vi "TestingStraight.vi"() -> ()   [LabVIEW 2016]
uses:
  <vilib>/Rock Robotics/WPI/Utilities/WPI_GetSetVariantRefNum.vi
panel:
  in  "Zero Yaw":bool
  in  "Config":T1={"Distance"=100.0, "MaxVelocity"=60.0, "MaxAccel"=50.0, "InitialVelocity"=0.0, "FinalVelocity"=0.0}
  out "Outputs":cluster{dbl, dbl, "Turn":dbl}(graph)
  in  "Go":bool
  in  "Go Backwards":bool
  out "Vel":cluster{dbl, "vel":dbl}(graph)
  out "Pos":cluster{dbl, "pos":dbl}(graph)={50.0, "pos"=48.31556625}
  in  "Linear Constants":T2={"FF"=0.0066, "AFF"=0.0018, "PID gains"={"P"=0.07, "I"=0.0, "D"=0.0}} {"PID gains"."D" format="%.3f"; "PID gains"."I" format="%.3f"; "PID gains"."P" format="%.3f"}
  # "MAKE DEFAULT"
  # ".009"
  # ".002"
  # ".07"
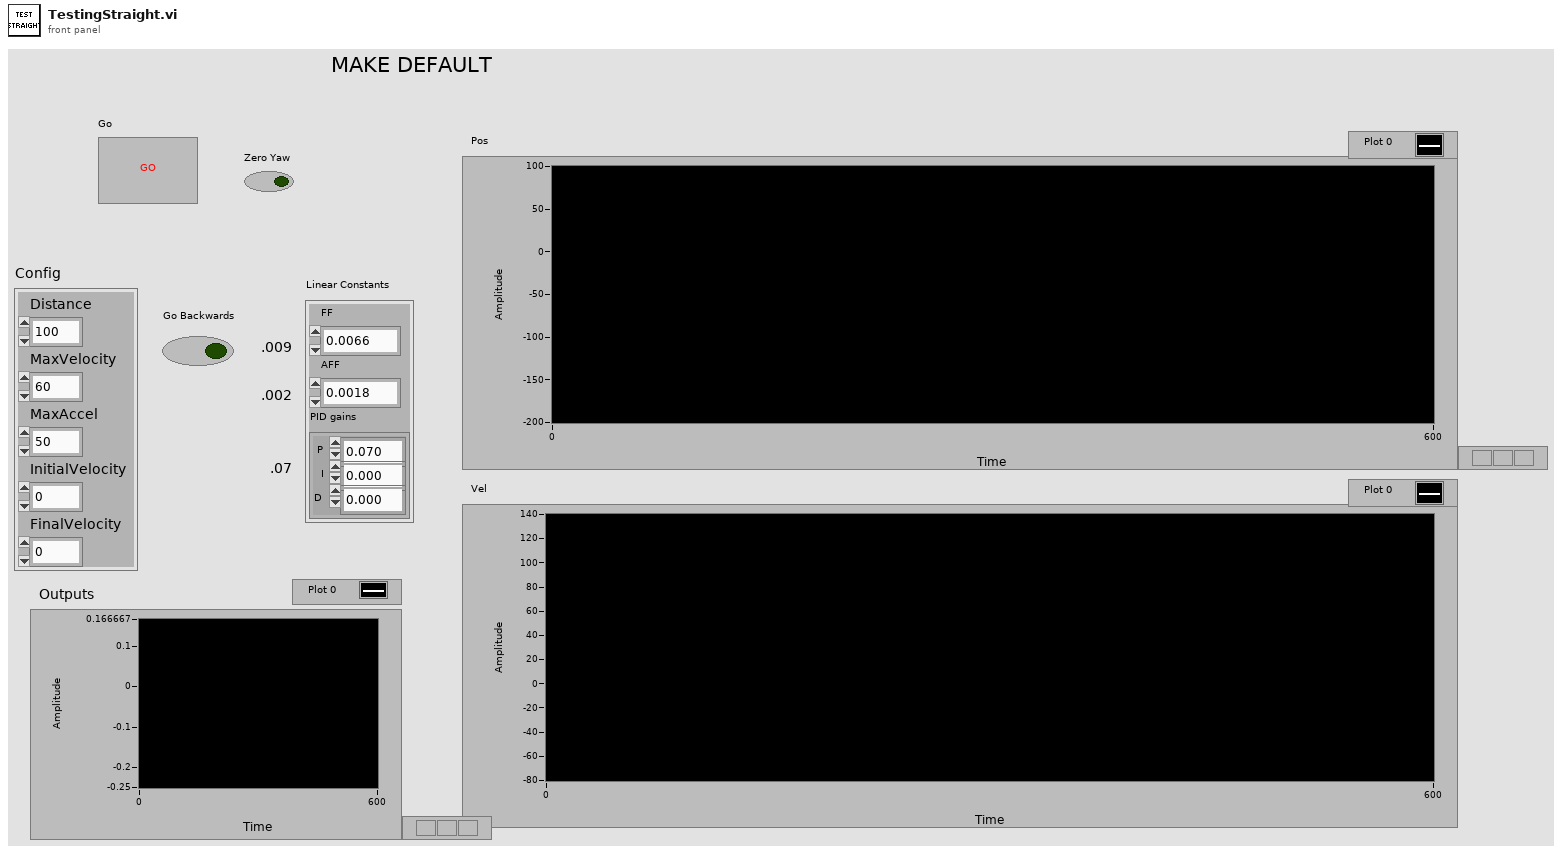
[diagram p1: front panel]
types:
  T1 = cluster{"Distance":dbl, "MaxVelocity":dbl, "MaxAccel":dbl, "InitialVelocity":dbl, "FinalVelocity":dbl}
  T2 = cluster{"FF":dbl, "AFF":dbl, "PID gains":cluster{"P":dbl, "I":dbl, "D":dbl}}
  T3 = typedef "WPI_EncoderDevRef.ctl" = cluster{"DevStatus":errorcluster, "EncoderIndex":T4, "CounterIndex":T5, "DistancePerCount":dbl, "Decoding Type":T6}
  T4 = typedef "FPGA_EncoderIdx.ctl" = enum8{"Enc 0", "Enc 1", "Enc 2", "Enc 3", "Enc 4", "Enc 5", "Enc 6", "Enc 7", "Invalid"}
  T5 = typedef "FPGA_CounterCtrSystemIndex.ctl" = enum8{"Ctr 0", "Ctr 1", "Ctr 2", "Ctr 3", "Ctr 4", "Ctr 5", "Ctr 6", "Ctr 7", "Invalid"}
  T6 = typedef "WPI_EncoderType.ctl" = enum16{"1x", "2x", "4x"}
  T7 = typedef "WPI_RobotDriveDevRef.ctl" = cluster{"DevStatus":errorcluster, "Motors[]":T8[], "Square Inputs":bool, "Max Output":dbl}
  T8 = typedef "WPI_MotorControlDeviceRef.ctl" = cluster{"DeviceStatus":errorcluster, "Type":T9, "PWM":cluster{"PWM Channel":T10, "DeadBand":T11}, "CAN":cluster{"Device Number":u8, "SetOutput VI Ref":variant, "GetOutput VI Ref":variant, "Enable VI Ref":variant, "Disable VI Ref":variant, "Data":variant}, "Invert":bool}
  T9 = typedef "WPI_MotorControlType.ctl" = enum16{"PWM", "CAN"}
  T10 = typedef "FPGA_DIOPWMChannel.ctl" = enum8{"PWM 0", "PWM 1", "PWM 2", "PWM 3", "PWM 4", "PWM 5", "PWM 6", "PWM 7", "PWM 8", "PWM 9", "PWM MXP 0", "PWM MXP 1", "PWM MXP 2", "PWM MXP 3", "PWM MXP 4", "PWM MXP 5", "PWM MXP 6", "PWM MXP 7", "PWM MXP 8", "PWM MXP 9", "Invalid"}
  T11 = typedef "WPI_PWMDeadband.ctl" = cluster{"Name":string, "maxPositivePwm":i32, "minPositivePwm":i32, "centerPwm":i32, "maxNegativePwm":i32, "minNegativePwm":i32, "angularRange":u16}
  T12 = cluster{dbl, "distance/rotation":dbl, "distance/rotation":dbl}
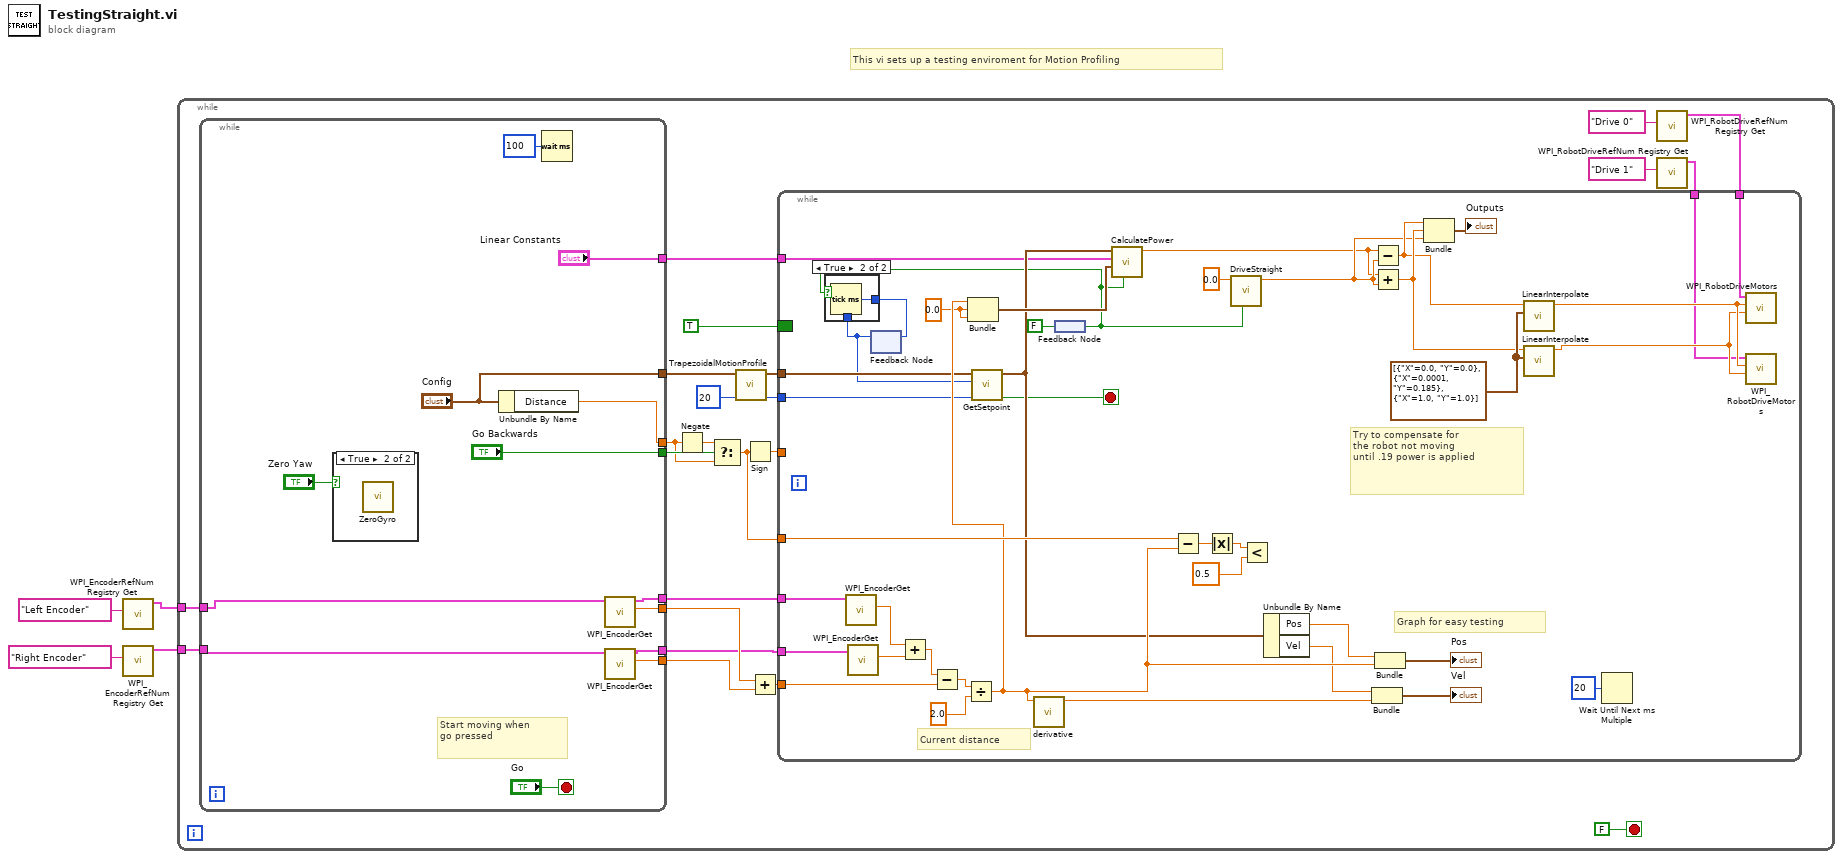
[diagram p0: block diagram]
diagram:
  # "This vi sets up a testing enviroment for Motion Profiling"
  n1 = call <vilib>:"WPI_EncoderRefNum Registry Get.vi"("refnum name"="Left Encoder") -> ("EncoderDevRef"=w2:T3)  [unwired: 9 in, 1 out]
  n2 = call <vilib>:"WPI_EncoderRefNum Registry Get.vi"("refnum name"="Right Encoder") -> ("EncoderDevRef"=w1:T3)  [unwired: 9 in, 1 out]
  n3 = while {
    tunnel: w2 -> [w15]
    tunnel: w1 -> [w14]
    stop <- FALSE stop-if-true
    n4 = while {
      tunnel: ["Go Backwards"] -> w16
      tunnel: w15 -> [w33]
      tunnel: w14 -> [w32]
      tunnel: [w37] -> w13
      tunnel: ["Config"] -> w12
      tunnel: ["Linear Constants"] -> w11
      tunnel: [w31] -> w8
      tunnel: [w30] -> w7
      tunnel: [w29] -> w6
      tunnel: [w28] -> w5
      stop <- "Go" stop-if-true
      # "Start moving when\ngo pressed"
      n5 = case shown="True" "Zero Yaw" {
        frame False {
        }
        frame True {
          n6 = call "ZeroGyro.vi"() -> ()  [unwired: 11 in, 1 out]
        }
      }
      n7 = Unbundle By Name("Config") -> ("Distance"=w37:dbl)
      n8 = Wait (ms)(milliseconds to wait=u32 100 ("millisecond multiple")) -> ()  [unwired: 1 out]
      n9 = call <vilib>:"WPI_EncoderGet.vi"("EncoderDevRef"=w33) -> ("Distance"=w30:dbl, "EncoderDevRef"=w29:T3)  [unwired: 5 in, 4 out]
      n10 = call <vilib>:"WPI_EncoderGet.vi"("EncoderDevRef"=w32) -> ("Distance"=w31:dbl, "EncoderDevRef"=w28:T3)  [unwired: 5 in, 4 out]
    }
    n11 = Negate(x=w13) -> (-x=w26:dbl)
    n12 = Select(t=w26, s=w16, f=w13) -> (s? t:f=w18:dbl)
    n13 = call "TrapezoidalMotionProfile.vi"("dt"=u32 20, "Config"=w12) -> ("dt"=w21:u32, "Profile"=w27:cluster{"Pos":dbl, "Vel":dbl, "Accel":dbl}[])  [unwired: 8 in]
    n14 = Sign(1:w18) -> (0:w17:dbl)
    n15 = Add(x=w7, y=w8) -> (x+y=w23:dbl)
    n16 = call <vilib>:"WPI_RobotDriveRefNum Registry Get.vi"("refnum name"="Drive 0") -> ("RobotDriveDevRef"=w10:T7)  [unwired: 9 in, 1 out]
    n17 = call <vilib>:"WPI_RobotDriveRefNum Registry Get.vi"("refnum name"="Drive 1") -> ("RobotDriveDevRef"=w9:T7)  [unwired: 9 in, 1 out]
    n18 = while {
      tunnel: w27 -> [w65]
      tunnel: w18 -> [w75]
      border: TRUE ("Reset") -> [_]
      tunnel: w23 -> [w70]
      tunnel: w21 -> [w64]
      tunnel: w6 -> [w57]
      tunnel: w5 -> [w56]
      tunnel: w17 -> [_]
      tunnel: w11 -> [w52]
      tunnel: w10 -> [w49]
      tunnel: w9 -> [w48]
      stop <- w58 stop-if-true
      w47 = cluster{"X":dbl, "Y":dbl}[] [{"X"=0.0, "Y"=0.0}, {"X"=0.0001, "Y"=0.185}, {"X"=1.0, "Y"=1.0}] ("Points")
      w67 = 0.0 ("distance/rotation")
      # "Try to compensate for\nthe robot not moving\nuntil .19 power is applied"
      # "Graph for easy testing"
      # "Current distance"
      n19 = call <vilib>:"WPI_EncoderGet.vi"("EncoderDevRef"=w57) -> ("Distance"=w73:dbl)  [unwired: 5 in, 5 out]
      n20 = call <vilib>:"WPI_EncoderGet.vi"("EncoderDevRef"=w56) -> ("Distance"=w53:dbl)  [unwired: 5 in, 5 out]
      n21 = feedback #1() -> (w50:u32)  [unwired: 1 in]
      n22 = Add(x=w73, y=w53) -> (x+y=w71:dbl)
      n23 = Subtract(x=w71, y=w70) -> (x-y=w72:dbl)
      n24 = Divide(x=w72, y=2.0 ("distance/rotation")) -> (x/y=w68:dbl)
      n25 = Bundle(w68, "distance/rotation"=w67, "distance/rotation"=w67) -> (w69:T12)  [unwired: 1 in]
      n26 = call "GetSetpoint.vi"("dt"=w64, "Start Time"=w50, "Profile"=w65) -> ("Profile done?"=w58:bool, "Setpoints"=w63:cluster{"Pos":dbl, "Vel":dbl, "Accel":dbl})  [unwired: 7 in]
      n27 = call "derivative.vi"("x"=w68) -> ("dx/dt"=w74:dbl)  [unwired: 10 in]
      n28 = feedback-in #2(FALSE ("Reset")) -> ()
      n29 = feedback #2() -> (w46:bool)
      n30 = case shown="True" w46 {
        tunnel: [w82 w83] -> w51
        tunnel: w50 -> [w82 _]
        frame False {
        }
        frame True {
          n31 = Tick Count (ms)() -> (millisecond timer value=w83:u32)
        }
      }
      n32 = feedback-in #1(w51) -> ()
      n33 = call "CalculatePower.vi"("Reset"=w46, "Process Variables"=w69, "Constants"=w52, "Setpoints"=w63) -> ("Power"=w41:dbl)  [unwired: 7 in]
      n34 = Subtract(x=w75, y=w68) -> (x-y=w79:dbl)
      n35 = Absolute Value(x=w79) -> (abs(x)=w78:dbl)
      n36 = call "DriveStraight.vi"("Reset"=w46, "Angle"=0.0) -> ("Turn"=w42:dbl)  [unwired: 9 in]
      n37 = Less?(x=w78, y=0.5 ("Closeness at end")) -> ()  [unwired: 1 out]
      n38 = Unbundle By Name(w63) -> ("Pos"=w62:dbl, "Vel"=w61:dbl)
      n39 = Bundle("Vel"=w61, "dx/dt"=w74) -> (→"Vel":cluster{"Vel":dbl, "dx/dt":dbl})  [unwired: 1 in]
      n40 = Subtract(x=w41, y=w42) -> (x-y=w43:dbl)
      n41 = Add(x=w41, y=w42) -> (x+y=w44:dbl)
      n42 = Bundle("Pos"=w62, w68) -> (→"Pos":cluster{"Pos":dbl, dbl})  [unwired: 1 in]
      n43 = Bundle(w43, w44, "Turn"=w42) -> (→"Outputs":cluster{dbl, dbl, "Turn":dbl})  [unwired: 1 in]
      n44 = call "LinearInterpolate.vi"("Points"=w47, "Value"=w43) -> ("Output"=w55:dbl)  [unwired: 9 in]
      n45 = call "LinearInterpolate.vi"("Points"=w47, "Value"=w44) -> ("Output"=w54:dbl)  [unwired: 9 in]
      n46 = Wait Until Next ms Multiple(millisecond multiple=u32 20) -> ()  [unwired: 1 out]
      n47 = call <vilib>:"WPI_RobotDriveMotors.vi"("RightSpeed"=w54, "LeftSpeed"=w55, "RobotDriveDevRef"=w49) -> ()  [unwired: 6 in, 3 out]
      n48 = call <vilib>:"WPI_RobotDriveMotors.vi"("RightSpeed"=w54, "LeftSpeed"=w55, "RobotDriveDevRef"=w48) -> ()  [unwired: 6 in, 3 out]
    }
  }
